vi "DATOS_VECTOR.vi"(1 "dato nuevo":string, 2 "entrada":string[](array[string])) -> (0 "salida":string[](array[string]))   [LabVIEW 2020]
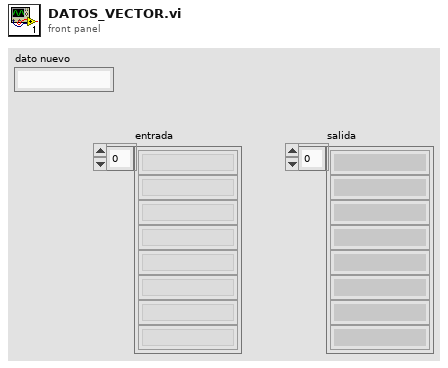
[diagram p1: front panel]
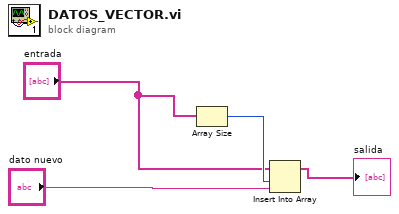
[diagram p0: block diagram]
diagram:
  n1 = Array Size(array="entrada") -> (size(s)=w4:i32)
  n2 = Insert Into Array(array="entrada", index=w4, new element="dato nuevo") -> (→"salida":string[])
